vi "InitSub.vi"(11 "SubChannel in":refnum<class "SubChannelCPU.lvclass">) -> (3 "SubChannel out":refnum<class "SubChannelCPU.lvclass">)   [LabVIEW 2019, in "MessengerM.lvlib" / "SubChannelCPU.lvclass"]
uses:
  SubChannelCPU.lvclass
  <resource>/ChannelSupport/_ChannelSupport/PipeLogic2/PipeLogic2.lvclass
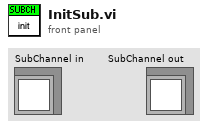
[diagram p1: front panel]
types:
  T1 = typedef "MessengerM.lvlib/Element.ctl" = string
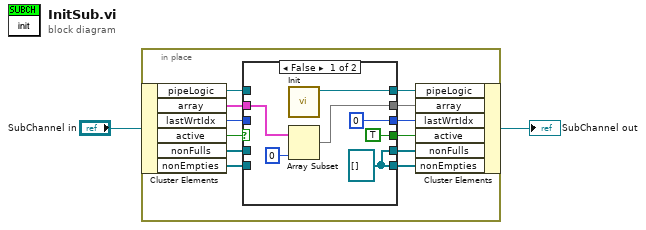
[diagram p0: block diagram]
diagram:
  n1 = in-place {
    n2 = in-place-cluster #1("SubChannel in") -> ("pipeLogic"=w7:refnum<class "PipeLogic2.lvclass">, "array"=w10:cluster{"elt":T1}[], "lastWrtIdx"=w11:i32, "active"=w14:bool, "nonFulls"=w4:refnum<k4>[], "nonEmpties"=w3:refnum<k4>[])
    n3 = case shown="False" w14 {
      selector: w14 -> [_ w27]
      tunnel: [TRUE w27] -> w13
      tunnel: [0 ("lastWrtIdx") w26] -> w12
      tunnel: w11 -> [_ w26]
      tunnel: w10 -> [w17 w25]
      tunnel: [w16 w25] -> w9
      tunnel: [w20 w24] -> w8
      tunnel: w7 -> [_ w24]
      tunnel: [w18 w23] -> w6
      tunnel: [w18 w22] -> w5
      tunnel: w4 -> [_ w23]
      tunnel: w3 -> [_ w22]
      frame False {
        w18 = refnum<k4>[] [] ("nonFulls")
        n4 = call <resource>:"Init.vi"() -> ("pipeLogic out"=w20:refnum<class "PipeLogic2.lvclass">)  [unwired: 11 in]
        n5 = Array Subset(array=w17, length=0) -> (w16:cluster{"elt":T1}[])  [unwired: 1 in]
      }
      frame True {
      }
    }
    n6 = in-place-cluster #1("pipeLogic"=w8, "array"=w9, "lastWrtIdx"=w12, "active"=w13, "nonFulls"=w6, "nonEmpties"=w5) -> (→"SubChannel out":refnum<class "SubChannelCPU.lvclass">)
  }
